vi "10_NOV_VARY_V.vi"() -> ()   [LabVIEW 2020]
uses:
  <instrlib>/Agilent B2900 Series/Agilent B2900 Series.lvlib
panel:
  out "Waveform Chart":dbl(graph)
  in  "Stop Button":bool
  out "Measured Current (Amp)":dbl
  in  "SELECT DEVICE":refnum<visa-resource-name>="USB0::0x0957::0x8E18::MY51140695::INSTR"
  in  "Channel":enum16{"Not Selected", "1", "2"}(ring)
  in  "Voltage(V)":dbl(slide) scale=0.0..0.1
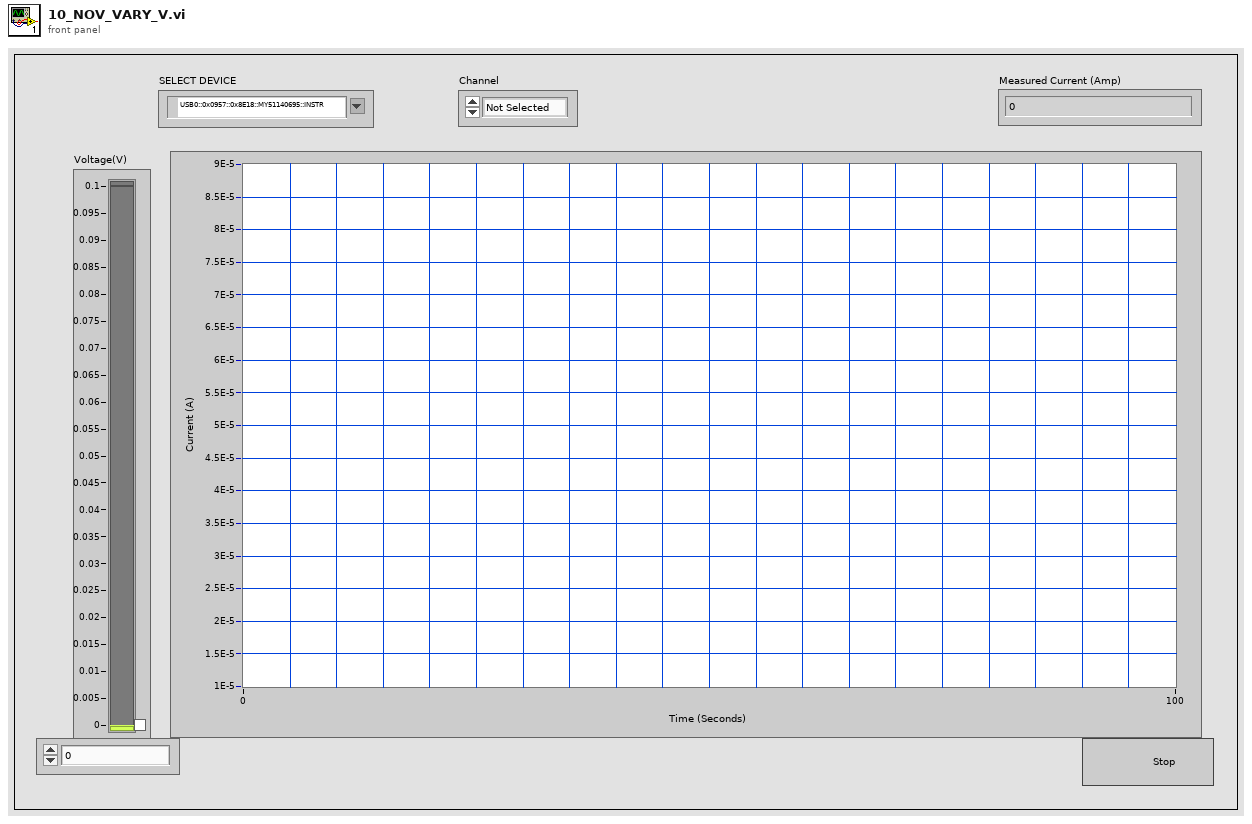
[diagram p1: front panel]
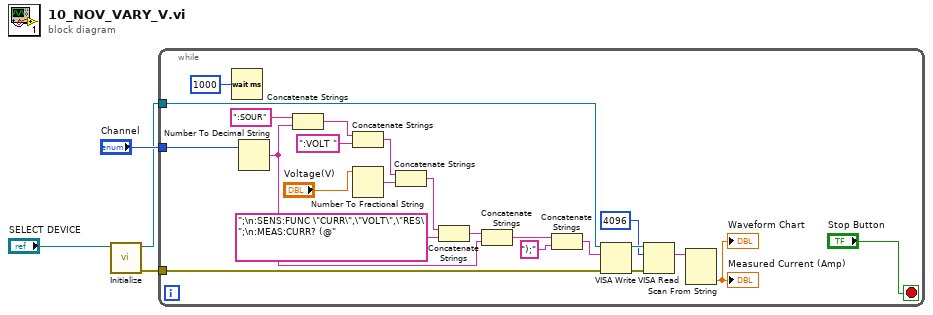
[diagram p0: block diagram]
diagram:
  n1 = call <instrlib>:"Initialize.vi"("VISA resource name"="SELECT DEVICE") -> ("error out"=w1:errorcluster, "VISA resource name out"=w2:refnum<visa-resource-name>)  [unwired: 9 in]
  n2 = while {
    tunnel: "Channel" -> [w25]
    tunnel: w2 -> [w14]
    tunnel: w1 -> [w13]
    stop <- "Stop Button" stop-if-true
    n3 = Wait (ms)(milliseconds to wait=u32 1000) -> ()  [unwired: 1 out]
    n4 = Number To Decimal String(number=w25) -> (decimal integer string=w18:string)  [unwired: 1 in]
    n5 = Concatenate Strings(":SOUR", w18) -> (w17:string)
    n6 = Concatenate Strings(w17, ":VOLT ") -> (w15:string)
    n7 = Number To Fractional String(number="Voltage(V)") -> (F-format string=w26:string)  [unwired: 3 in]
    n8 = Concatenate Strings(w15, w26) -> (w24:string)
    n9 = Concatenate Strings(w24, ";\n:SENS:FUNC \"CURR\",\"VOLT\",\"RES\";\n:MEAS:CURR? (@") -> (w22:string)
    n10 = Concatenate Strings(w22, w18) -> (w21:string)
    n11 = Concatenate Strings(w21, ");" ("string")) -> (w12:string)
    n12 = VISA Write(VISA resource name=w14, write buffer=w12, error in (no error)=w13) -> (VISA resource name out=w11:refnum<visa-resource-name>, error out=w10:errorcluster)  [unwired: 1 out]
    n13 = VISA Read(VISA resource name=w11, byte count=u32 4096, error in (no error)=w10) -> (read buffer=w6:string)  [unwired: 3 out]
    n14 = Scan From String(input string=w6) -> (output 1=→"Measured Current (Amp)" →"Waveform Chart":dbl)  [unwired: 4 in, 3 out]
  }
